vi "RT-State-FGV.vi"(6 "error in":errorcluster, 8 "RT-States in":T1, 9 "Mode":enum16{"Write", "Read", "Read-Clear"}(ring)=enum."Read") -> (0 "error out":errorcluster, 2 "NewVal?":bool, 3 "RT-States out":T1)   [LabVIEW 2016]
uses:
  RT-Typedefinitions/RT-States.ctl
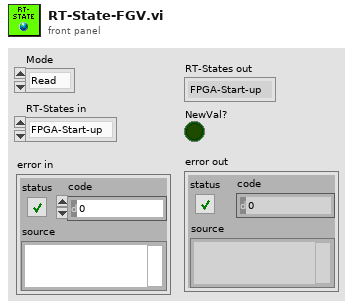
[diagram p1: front panel]
types:
  T1 = typedef "RT-States.ctl" = enum8{"FPGA-Start-up", "IDLE", "Set-IRQ", "Capture", "Save", "Error"}
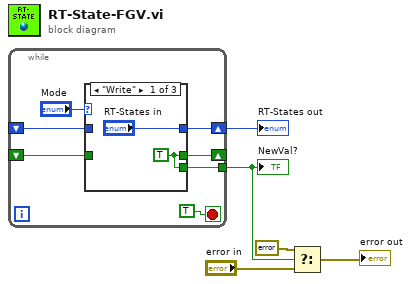
[diagram p0: block diagram]
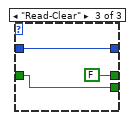
[diagram p3: hidden frame]
diagram:
  n1 = while {
    shift-right: [w11] -> w5
    shift-left: _ -> [w10]
    shift-right: [w8] -> _
    shift-left: _ -> [w7]
    tunnel: [w6] -> w2
    stop <- TRUE stop-if-true
    n2 = case shown="\"Write\"" "Mode" {
      tunnel: ["RT-States in" w16 w19] -> w11
      tunnel: w10 -> [_ w16 w19]
      tunnel: [w13 w15 FALSE] -> w8
      tunnel: w7 -> [_ w15 w17]
      tunnel: [w13 w15 w17] -> w6
      frame "Write" {
        w13 = TRUE
      }
      frame "Read", Default {
      }
      frame "Read-Clear" {
      }
    }
  }
  "RT-States out" <- w5
  "NewVal?" <- w2
  n3 = Select(t=errorcluster {"status"=FALSE, "code"=0, "source"=""} ("f"), s=w2, f="error in") -> (s? t:f=→"error out":errorcluster)
